vi "23384_Davis_Poku_Amankwa_Amankwa.DavisPoku.MNE1201.1.5_348252_1905103444.vi"() -> ()   [LabVIEW 2018]
panel:
  out "Balance(B)":dbl
  in  "No of years (N)":dbl
  in  "Interest (I)":dbl
  in  "Principal  (P)":dbl
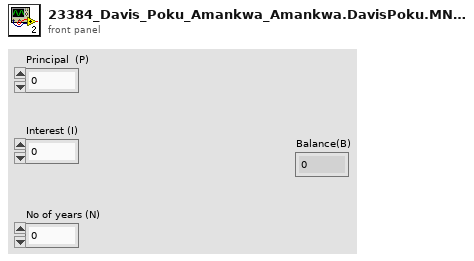
[diagram p1: front panel]
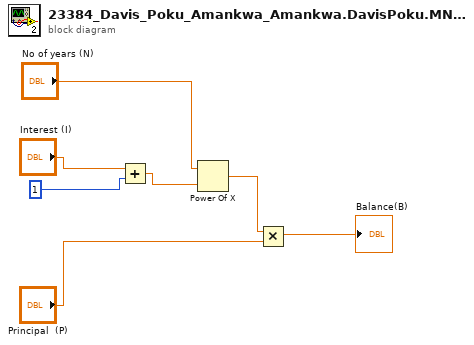
[diagram p0: block diagram]
diagram:
  n1 = Add(x="Interest (I)", y=1) -> (x+y=w5:dbl)
  n2 = Power Of X(1:w5, 2:"No of years (N)") -> (0:w2:dbl)
  n3 = Multiply(x=w2, y="Principal  (P)") -> (x*y=→"Balance(B)":dbl)
